vi "test_host.vi"() -> ()   [LabVIEW 2014]
uses:
  <vilib>/FPGAPlugInAG/PXIe-7962R/niLvFpga_Open_PXIe-7962R.vi
  <vilib>/rvi/interface/common/dynamic/niFpgaDynamicAddResources.vi
  <vilib>/LabVIEW Targets/FPGA/FlexRIO/CustomFPGAMethods/79XXR_Method_IOModuleStatusImpl.vi
  <vilib>/Utility/error.llb/Error Cluster From Error Code.vi
  <vilib>/rvi/errors/niLvFpgaAdjustHostInterfaceError.vi
  <vilib>/rvi/interface/common/niFpgaWaitOnOcc.vi
  <instrlib>/_niInstr/Streaming/v1/Host/Public/Start Finite Stream.vi
  <instrlib>/niSync/niSync.llb/niSync Initialize (IVI).vi
  <instrlib>/_niInstr/Streaming/v1/Host/Public/Wait for Stream.vi
  <vilib>/FPGAPlugInAG/Dynamic/niLvFpga_Close_Dynamic.vi
  <vilib>/rvi/interface/nirviOpenFPGA/nirviOpenFPGA.xnode
  FPGA Bitfiles/MochiFPGAControl_FPGATarget_pxie7962fpga_XsUx6Pt6QBg.lvbitx
  <vilib>/rvi/interface/nirviMethod/nirviMethod.xnode
  <vilib>/rvi/interface/nirviReadWriteControl/nirviReadWriteControl.xnode
  <vilib>/rvi/interface/nirviCloseFPGA/nirviCloseFPGA.xnode
  <instrlib>/_niInstr/Streaming/v1/Host/niInstr Streaming v1 Host.lvlib
  <vilib>/rvi/errors/niLvFpgaMergeErrorWithErrorCode.vi
  <vilib>/rvi/interface/Simulation/niFpgaSimulationCallBeginRW.vi
  NiFpgaLv.dll
  <vilib>/FPGAPlugInAG/Dynamic/niLvFpga_ConfigureFifo_Dynamic.vi
  <vilib>/FPGAPlugInAG/Dynamic/niLvFpga_StartFifo_Dynamic.vi
  <vilib>/FPGAPlugInAG/Dynamic/niLvFpga_ReadFifo_Dynamic.vi
panel:
  out "Bits out DRAM":u64
  out "Writes to DRAM":u64
  in  "?":enum32{"AI 0", "All AI"}(tab)
  out "AI 0":dbl[](graph)
  out "All AI":dbl[][](graph)
  in  "Debug":bool
  out "Bits out DMA":u64
  out "Bits aquired":u64
  out "Writes to DMA":u64
  out "Samples Aquired":u64
  out "Voltage":dbl[][](array[numeric])
  out "Counts":i16[][](array[numeric])
  out "error out":errorcluster
  out "samples transferred":u64
  in  "stop":bool
  out "Raw DMA readout":u64[](array[numeric])
  in  "num samples":u64=40000
  in  "Go":bool
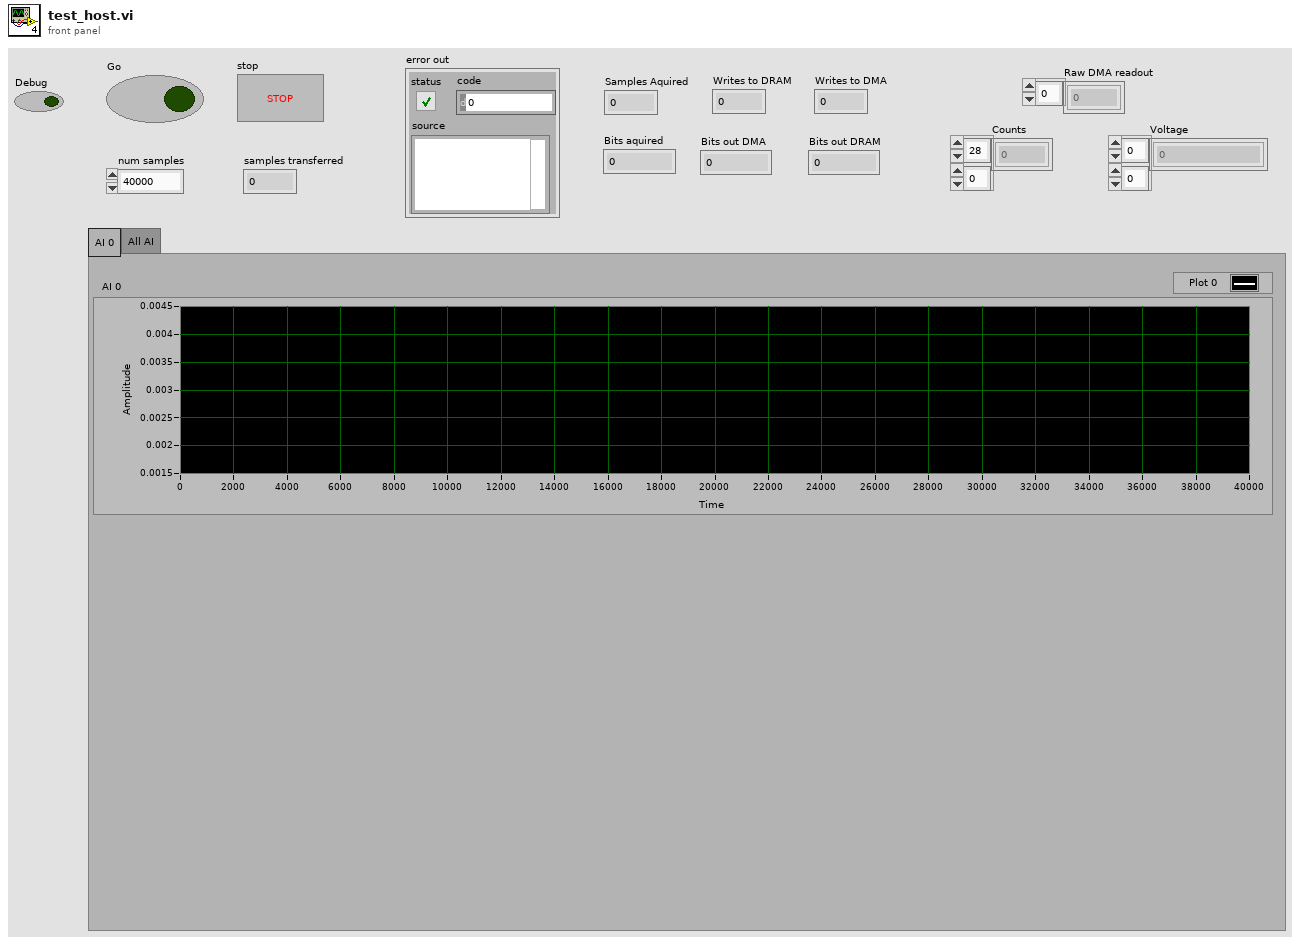
[diagram p1: front panel]
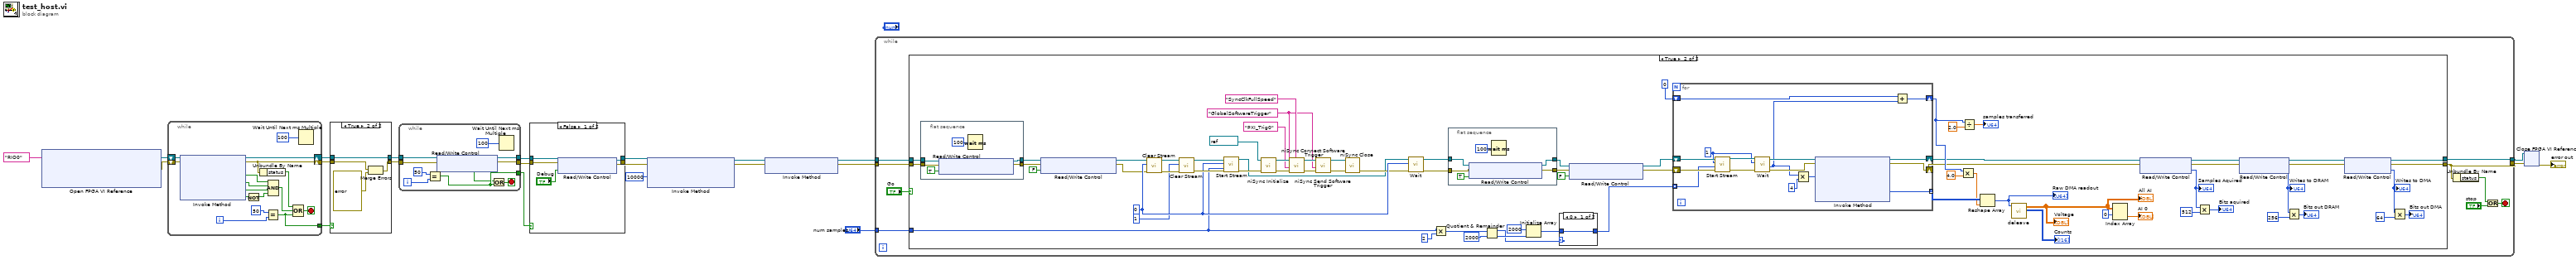
[diagram p0: block diagram]
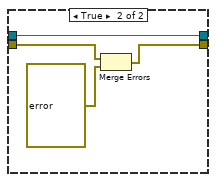
[diagram p2: hidden frame]
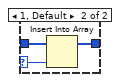
[diagram p5: hidden frame]
diagram:
  n1 = xnode "Open FPGA VI Reference"("resource name"=tag "RIO0") -> ("FPGA VI Reference Out"=w4:refnum<k20>, "error out"=w5:errorcluster)  [unwired: 1 in]
  n2 = while {
    shift-right: [w29] -> w12
    shift-left: w5 -> [w37]
    shift-right: [w36] -> w10
    shift-left: w4 -> [w38]
    tunnel: [w25] -> w11
    i -> [w31]
    stop <- w26 stop-if-true
    n3 = xnode "Invoke Method"("FPGA VI Reference In"=w38, "error in"=w37) -> ("FPGA VI Reference Out"=w36:refnum<k20>, "error out"=w29:errorcluster, "IO Module Present?"=w35:bool, "Power Enabled?"=w34:bool, "IO Enabled?"=w33:bool, "IO Module Mismatch?"=w24:bool)
    n4 = Not(x=w24) -> (.not. x?=w23:bool)
    n5 = Unbundle By Name(w29) -> ("status"=w28:bool)
    n6 = Equal?(x=50, y=w31) -> (x = y?=w25:bool)
    n7 = Compound Arithmetic op=AND(w35, w34, w33, w23) -> (w27:bool)
    n8 = Compound Arithmetic op=OR(w28, w27, w25) -> (w26:bool)
    n9 = Wait Until Next ms Multiple(millisecond multiple=u32 100) -> ()  [unwired: 1 out]
  }
  n10 = case shown="True" w11 {
    tunnel: w12 -> [w39 w43]
    tunnel: [w39 w42] -> w8
    tunnel: w10 -> [w40 w41]
    tunnel: [w40 w41] -> w9
    frame False {
    }
    frame True {
      n11 = Merge Errors(w43, errorcluster {"status"=TRUE, "code"=-1, "source"="The IO Module was not present, powered, or the IO were not enabled.  Verify the NI 5752 is securly connected and try again."} ("error in")) -> (w42:errorcluster)
    }
  }
  n12 = while {
    tunnel: w9 -> [w49]
    tunnel: [w46] -> w2
    tunnel: [w47] -> w1
    tunnel: [w50] -> w3
    tunnel: w8 -> [w48]
    i -> [w53]
    stop <- w51 stop-if-true
    n13 = Equal?(x=50, y=w53) -> (x = y?=w50:bool)
    n14 = xnode "Read/Write Control"("FPGA VI Reference In"=w49, "error in"=w48) -> ("FPGA VI Reference Out"=w46:refnum<k20>, "error out"=w47:errorcluster, "IO Module Init Done"=w45:bool)
    n15 = Or(x=w45, y=w50) -> (x .or. y?=w51:bool)
    n16 = Wait Until Next ms Multiple(millisecond multiple=u32 100) -> ()  [unwired: 1 out]
  }
  n17 = case shown="False" w3 {
    tunnel: w1 -> [w56 w62]
    tunnel: [w55 w61] -> w6
    tunnel: w2 -> [w59 w60]
    tunnel: [w58 w60] -> w7
    frame False {
      n18 = xnode "Read/Write Control"("FPGA VI Reference In"=w59, "error in"=w56, "Output Debug Data"="Debug") -> ("FPGA VI Reference Out"=w58:refnum<k20>, "error out"=w55:errorcluster)
    }
    frame True {
      n19 = Merge Errors(w62, errorcluster {"status"=TRUE, "code"=-1, "source"="The IO Module CLIP was not ready. If you are using any external clocks, make sure they are connected and within the supported specifications."} ("error in")) -> (w61:errorcluster)
    }
  }
  n20 = xnode "Invoke Method"("FPGA VI Reference In"=w7, "error in"=w6, "Requested Depth"=u32 10000) -> ("FPGA VI Reference Out"=w21:refnum<k20>, "error out"=w20:errorcluster)  [unwired: 1 out]
  n21 = xnode "Invoke Method"("FPGA VI Reference In"=w21, "error in"=w20) -> ("FPGA VI Reference Out"=w19:refnum<k20>, "error out"=w18:errorcluster)
  n22 = while {
    tunnel: w19 -> [w71]
    tunnel: w18 -> [w67]
    tunnel: "num samples" -> [w70]
    tunnel: [w69] -> w14
    tunnel: [w66] -> w16
    stop <- w68 stop-if-true
    n23 = case shown="True" "Go" {
      tunnel: w71 -> [w74 w122]
      tunnel: w70 -> [_ w99]
      tunnel: [w74 w90] -> w69
      tunnel: w67 -> [w73 w89]
      tunnel: [w73 w88] -> w66
      frame False {
        (unwired) errorcluster {"status"=FALSE, "code"=0, "source"=""} ("error out")
      }
      frame True {
        w76 = "GlobalSoftwareTrigger" ("source terminal")
        w140 = 0 ("stream index")
        n24 = flat-sequence {
          tunnel: [w175] -> w126
          tunnel: w122 -> [w174]
          tunnel: [w173] -> w121
          tunnel: w89 -> [w172]
          frame #0 {
            n25 = xnode "Read/Write Control"("FPGA VI Reference In"=w174, "error in"=w172, "Reset DRAM write address"=TRUE) -> ("FPGA VI Reference Out"=w173:refnum<k20>, "error out"=w175:errorcluster)
            n26 = Wait (ms)(milliseconds to wait=u32 100) -> ()  [unwired: 1 out]
          }
        }
        n27 = xnode "Read/Write Control"("FPGA VI Reference In"=w121, "error in"=w126, "Reset DRAM write address"=FALSE) -> ("FPGA VI Reference Out"=w100:refnum<k20>, "error out"=w106:errorcluster)
        n28 = call <instrlib>:"Clear Stream.vi"("error in (no error)"=w106, "stream index"=w140, "refnum in"=w100) -> ("error out"=w144:errorcluster, "refnum out"=w145:refnum<k20>)  [unwired: 7 in]
        n29 = call <instrlib>:"Clear Stream.vi"("error in (no error)"=w144, "stream index"=1, "refnum in"=w145) -> ("error out"=w142:errorcluster, "refnum out"=w143:refnum<k20>)  [unwired: 7 in]
        n30 = call-poly <instrlib>:"Start Stream.vi"("error in (no error)"=w142, "num samples"=w99, "stream index"=w140, "refnum in"=w143) -> ("error out"=w83:errorcluster, "refnum out"=w75:refnum<k20>)  [unwired: 6 in]
        n31 = call-poly <instrlib>:"niSync Initialize.vi"("error in (no error)"=w83, "resource name"=refnum<k15> "Sync0") -> ("error out"=w87:errorcluster, "instrument handle out"=w86:refnum<k15>)  [unwired: 8 in]
        n32 = call <instrlib>:"niSync Connect Software Trigger.vi"("synchronization clock"="SyncClkFullSpeed", "error in (no error)"=w87, "destination terminal"="PXI_Trig0", "source terminal"=w76, "instrument handle"=w86) -> ("error out"=w85:errorcluster, "instrument handle out"=w84:refnum<k15>)  [unwired: 5 in]
        n33 = call <instrlib>:"niSync Send Software Trigger.vi"("error in (no error)"=w85, "source terminal"=w76, "instrument handle"=w84) -> ("error out"=w81:errorcluster, "instrument handle out"=w82:refnum<k15>)  [unwired: 7 in]
        n34 = call <instrlib>:"niSync Close.vi"("error in (no error)"=w81, "instrument handle"=w82) -> ("error out"=w80:errorcluster)  [unwired: 9 in]
        n35 = call-poly <instrlib>:"Wait.vi"("error in (no error)"=w80, "stream index"=w140, "refnum in"=w75) -> ("error out"=w123:errorcluster, "refnum out"=w120:refnum<k20>)  [unwired: 5 in, 2 out]
        n36 = Multiply(x=w99, y=u64 2) -> (x*y=w112:u64)
        n37 = flat-sequence {
          tunnel: w123 -> [w170]
          tunnel: [w168] -> w124
          tunnel: w120 -> [w167]
          tunnel: [w166] -> w119
          frame #0 {
            n38 = xnode "Read/Write Control"("FPGA VI Reference In"=w167, "error in"=w170, "Reset DRAM read address"=TRUE ("Reset DRAM write address")) -> ("FPGA VI Reference Out"=w166:refnum<k20>, "error out"=w168:errorcluster)
            n39 = Wait (ms)(milliseconds to wait=u32 100) -> ()  [unwired: 1 out]
          }
        }
        n40 = Quotient & Remainder(x=w112, y=u64 2000) -> (x-y*floor(x/y)=w101:u64, floor(x/y)=w110:u64)
        n41 = Initialize Array(u64 2000 ("element"), w110) -> (w108:u64[])
        n42 = case shown="0" w101 {
          selector: w101 -> [_ w147]
          tunnel: w108 -> [w146 w149]
          tunnel: [w146 w148] -> w107
          frame 0 {
          }
          frame 1, Default {
            n43 = Insert Into Array(array=w149, new element=w147) -> (w148:u64[])  [unwired: 1 in]
          }
        }
        n44 = xnode "Read/Write Control"("FPGA VI Reference In"=w119, "error in"=w124, "Reset DRAM read address"=FALSE ("Reset DRAM write address")) -> ("FPGA VI Reference Out"=w113:refnum<k20>, "error out"=w114:errorcluster)
        n45 = for {
          shift-right: [w151] -> w105
          shift-left: w113 -> [w162]
          shift-right: [w150] -> w98
          shift-left: w114 -> [w161]
          shift-right: [w165] -> w116
          shift-left: u64 0 -> [w158]
          tunnel: w107 -> [w159] mode=indexing
          tunnel: [w152] -> w104 mode=indexing
          w160 = 1 ("stream index")
          n46 = call-poly <instrlib>:"Start Stream.vi"("error in (no error)"=w161, "num samples"=w159, "stream index"=w160, "refnum in"=w162) -> ("error out"=w163:errorcluster, "refnum out"=w164:refnum<k20>)  [unwired: 6 in]
          n47 = call-poly <instrlib>:"Wait.vi"("error in (no error)"=w163, "stream index"=w160, "refnum in"=w164) -> ("error out"=w156:errorcluster, "samples transferred"=w154:u64, "refnum out"=w157:refnum<k20>)  [unwired: 5 in, 1 out]
          n48 = Multiply(x=w154, y=u64 4) -> (x*y=w155:u64)
          n49 = xnode "Invoke Method"("FPGA VI Reference In"=w157, "error in"=w156, "Number of Elements"=w155) -> ("FPGA VI Reference Out"=w151:refnum<k20>, "error out"=w150:errorcluster, "Data"=w152:u64[])  [unwired: 1 in, 1 out]
          n50 = Add(x=w158, y=w154) -> (x+y=w165:u64)
        }
        n51 = Multiply(x=w116, y=4.0) -> (x*y=w103:dbl)
        n52 = Divide(x=w116, y=2.0) -> (x/y=→"samples transferred":dbl)
        n53 = Reshape Array(w104, w103) -> (w102:u64[])
        "Raw DMA readout" <- w102
        n54 = call "deleave.vi"("Data"=w102) -> ("Counts"=→"Counts":i16[][], "Voltage"=w129:dbl[][])  [unwired: 9 in]
        "Voltage" <- w129
        "All AI" <- w129
        n55 = Index Array(array=w129, index (row)=0) -> (element=→"AI 0":dbl[])  [unwired: 1 in]
        n56 = xnode "Read/Write Control"("FPGA VI Reference In"=w105, "error in"=w98) -> ("FPGA VI Reference Out"=w94:refnum<k20>, "error out"=w93:errorcluster, "Samples Aquired"=w136:u64)
        "Samples Aquired" <- w136
        n57 = Multiply(x=w136, y=u64 512) -> (x*y=→"Bits aquired":u64)
        n58 = xnode "Read/Write Control"("FPGA VI Reference In"=w94, "error in"=w93) -> ("FPGA VI Reference Out"=w92:refnum<k20>, "error out"=w91:errorcluster, "Writes to DRAM"=w96:u64)
        "Writes to DRAM" <- w96
        n59 = Multiply(x=w96, y=u64 256) -> (x*y=→"Bits out DRAM":u64)
        n60 = xnode "Read/Write Control"("FPGA VI Reference In"=w92, "error in"=w91) -> ("FPGA VI Reference Out"=w90:refnum<k20>, "error out"=w88:errorcluster, "Writes to DMA"=w133:u64)
        "Writes to DMA" <- w133
        n61 = Multiply(x=w133, y=u64 64) -> (x*y=→"Bits out DMA":u64)
      }
    }
    n62 = Unbundle By Name(w66) -> ("status"=w64:bool)
    n63 = Or(x=w64, y="stop") -> (x .or. y?=w68:bool)
  }
  n64 = xnode "Close FPGA VI Reference"("FPGA VI Reference In"=w14, "error in"=w16) -> ("error out"=→"error out":errorcluster)
